vi "X DIM conditions.Facade.vi"(0 "Data In":T7, 2 "Display State In":T5, 3 "Container State":T6) -> (6 "Data Out":T7, 7 "Display State Out":T5, 8 "Action":T4)   [LabVIEW 2014, in "X DIM conditions.xctl"]
uses:
  X DIM conditions.xctl
  X DIM conditions.Data.ctl
  PTSequencer/PTSequencer.DIM service condition.ctl
  CSCore/CSSystem/CoreDefs/CoreDefs.rawDataType.ctl
  <vilib>/_xctls/Container State.ctl
  X DIM conditions.State.ctl
  <vilib>/_xctls/Action.ctl
  CSCore/CSSystem/CoreLib/CoreLib.string 2 byte array.vi
  CSCore/CSSystem/CoreLib/CoreLib.int 2 byte array.vi
  CSCore/CSSystem/CoreLib/CoreLib.int array 2 byte array.vi
  CSCore/CSSystem/CoreLib/CoreLib.short 2 byte array.vi
  CSCore/CSSystem/CoreLib/CoreLib.short array 2 byte array.vi
  CSCore/CSSystem/CoreLib/CoreLib.double 2 byte array.vi
  CSCore/CSSystem/CoreLib/CoreLib.double array 2 byte array.vi
  CSCore/CSSystem/CoreLib/CoreLib.float 2 byte array.vi
  CSCore/CSSystem/CoreLib/CoreLib.float array 2 byte array.vi
  <vilib>/_xctls/XControlSupport.lvlib
  CSCore/CSSystem/CoreLib/CoreLib.lvlib
  _common/PTUtils/PTUtils.lvlib
  CSlibraries/UtilityLib/UtilityLib.lvlib
  PTSequencer/PTSequencer.lvlib
panel:
  in  "element":T1
  in  "Scrollbar":i32(c297)
  in  "Control":T3
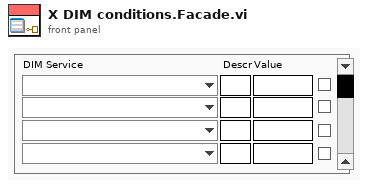
[diagram p1: front panel]
types:
  T1 = typedef "PTSequencer.lvlib/PTSequencer.DIM service condition.ctl" = cluster{"DIM service":string, "descr":string, "nomValue":T2, "actValue":T2, "matched":bool, "DIM Status":cluster{"no link":bool, "quality":i32, "Time Stamp":timestamp}}
  T2 = typedef "CoreDefs.rawDataType.ctl" = i8[]
  T3 = cluster{"Name 1":u16, "Descr 1":string, "Value 1":string, "Used 1":bool, "Name 2":u16, "Descr 2":string, "Value 2":string, "Used 2":bool, "Name 3":u16, "Descr 3":string, "Value 3":string, "Used 3":bool, "Name 4":u16, "Descr 4":string, "Value 4":string, "Used 4":bool}
  T4 = typedef "XControlSupport.lvlib/Action.ctl" = cluster{"Data Changed?":bool, "State Changed?":bool, "Action Name":string}
  T5 = typedef "X DIM conditions.xctl/X DIM conditions.State.ctl" = cluster{"index":i32}
  T6 = typedef "XControlSupport.lvlib/Container State.ctl" = cluster{"Indicator?":bool, "Run Mode?":bool, " Refnum":refnum<vi>}
  T7 = typedef "X DIM conditions.xctl/X DIM conditions.Data.ctl" = cluster{"DIM Services":string[], "data decsriptors":string[], "stop conditions":T1[]}
  T8 = enum8{"Enabled", "Disabled", "Disabled and Grayed Out"}
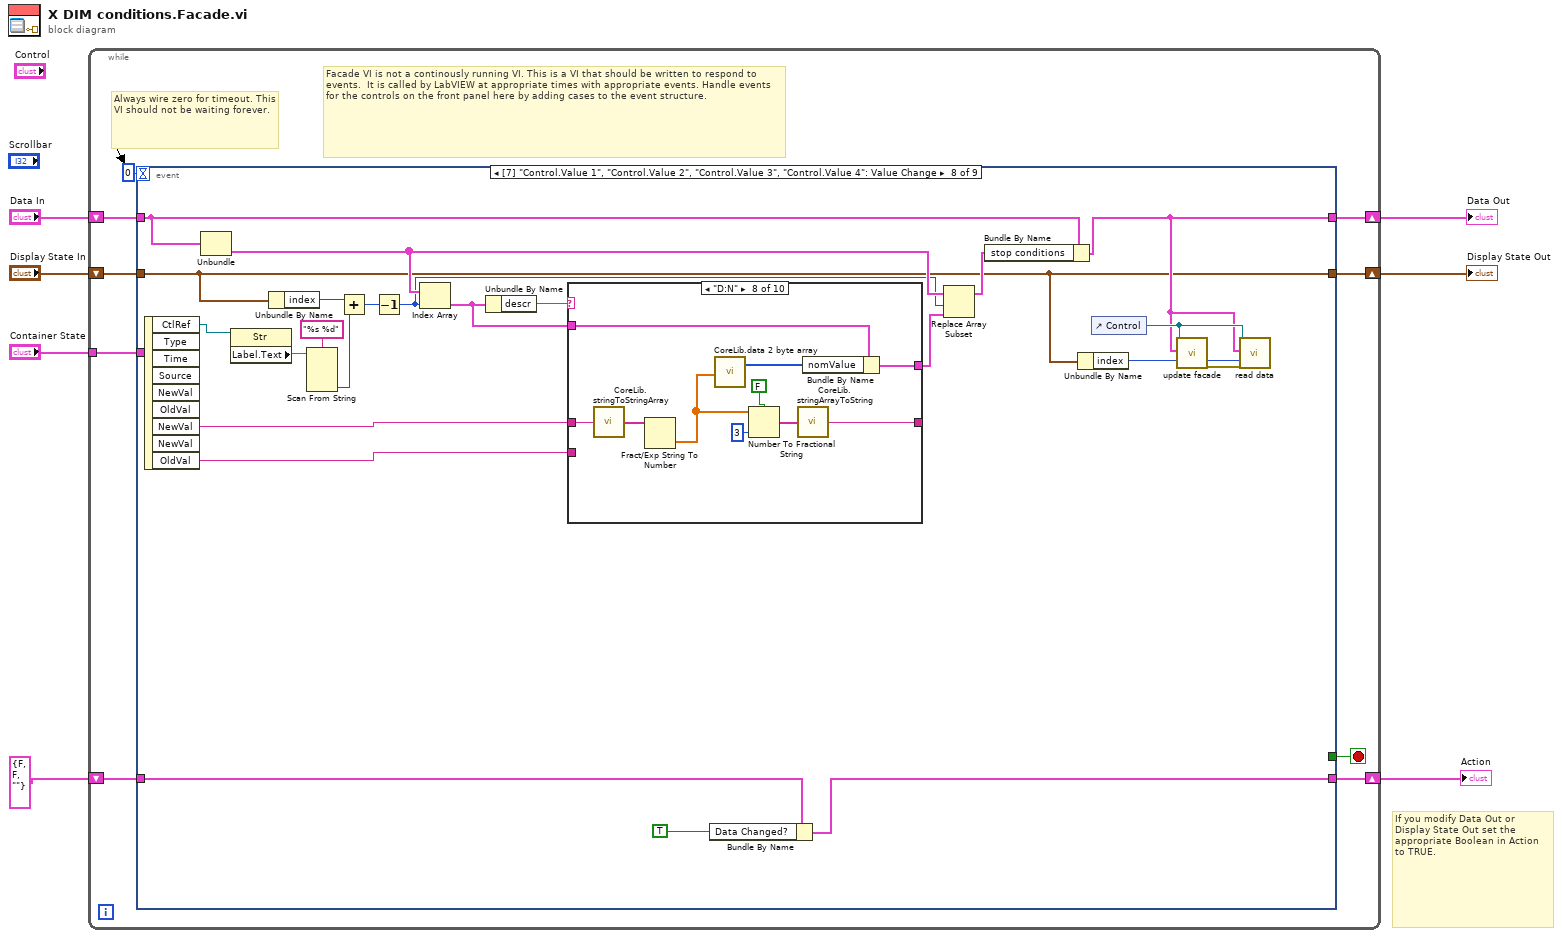
[diagram p0: block diagram]
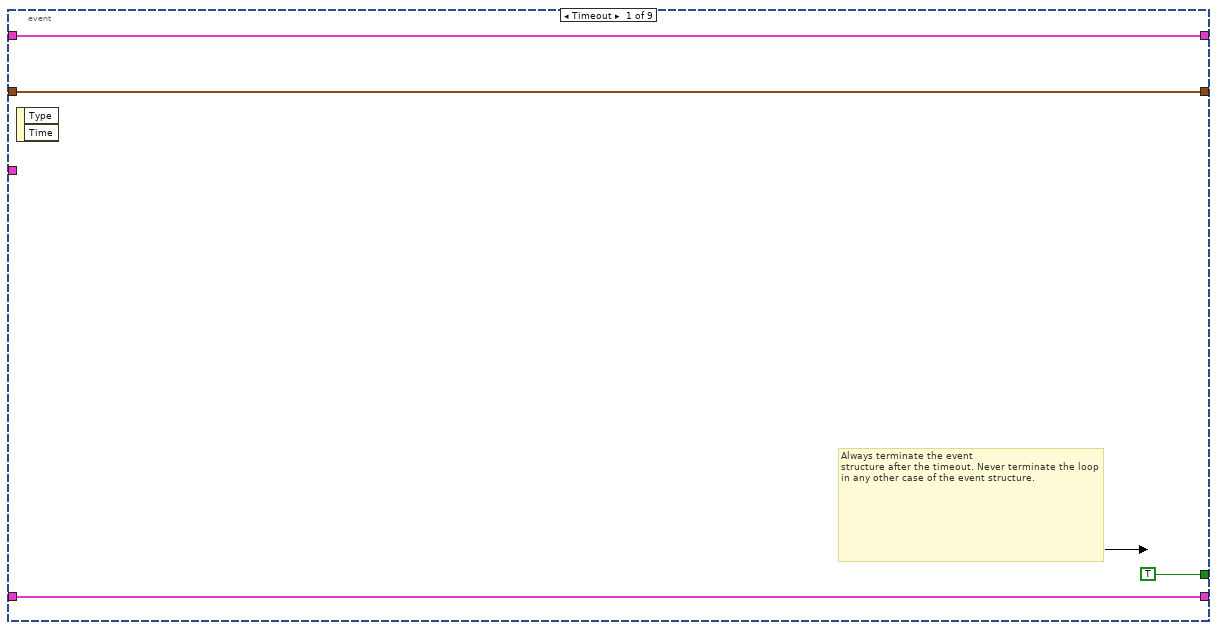
[diagram p2: hidden frame]
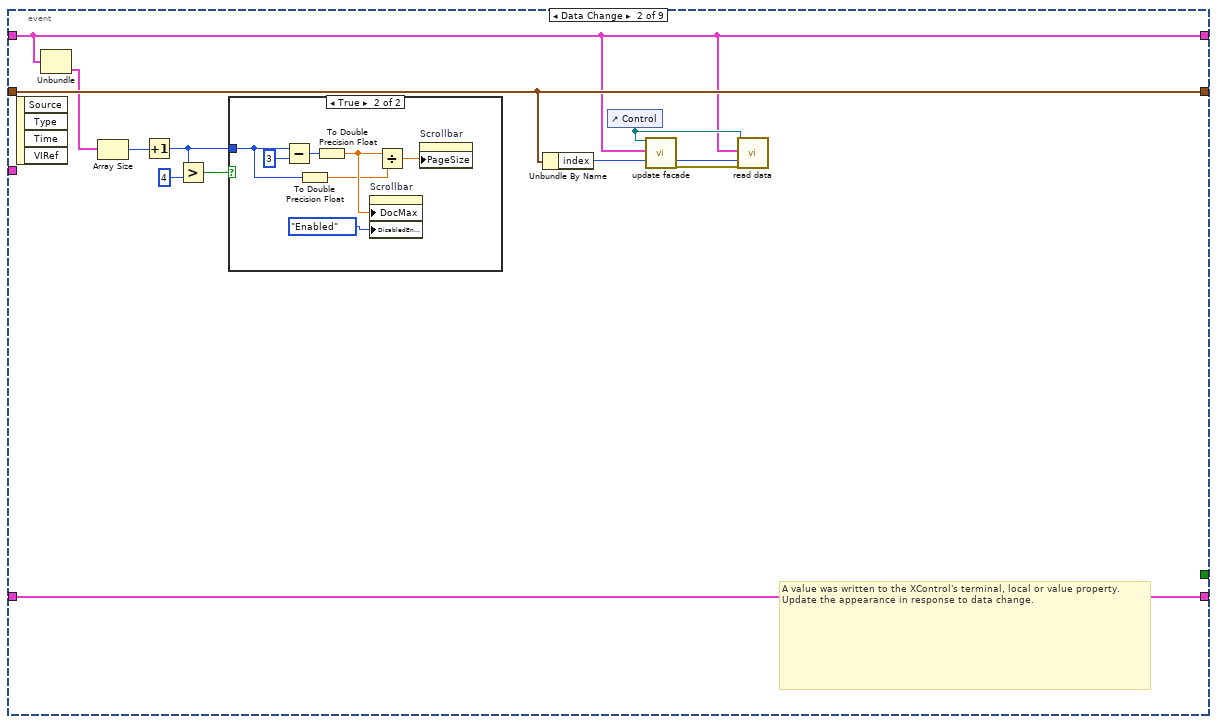
[diagram p3: hidden frame]
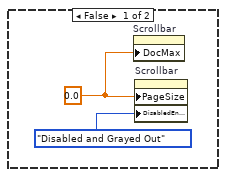
[diagram p4: hidden frame]
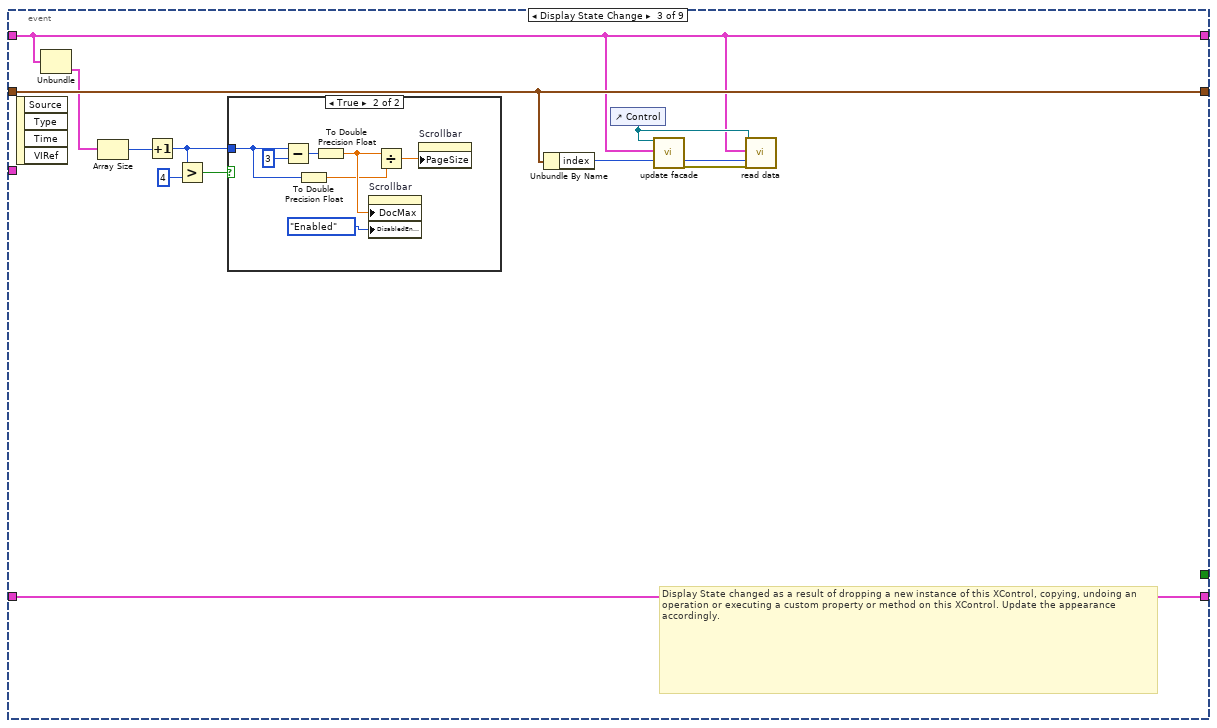
[diagram p5: hidden frame]
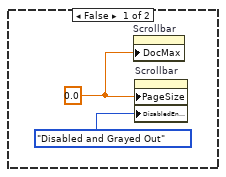
[diagram p6: hidden frame]
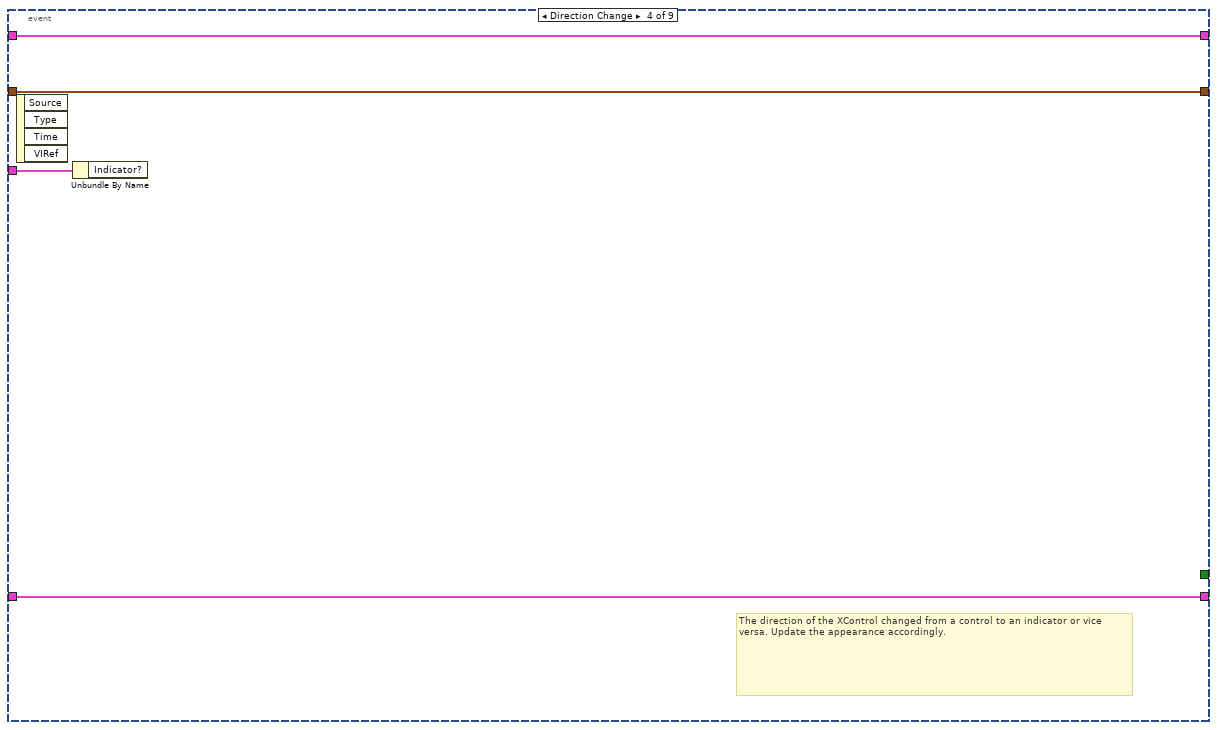
[diagram p7: hidden frame]
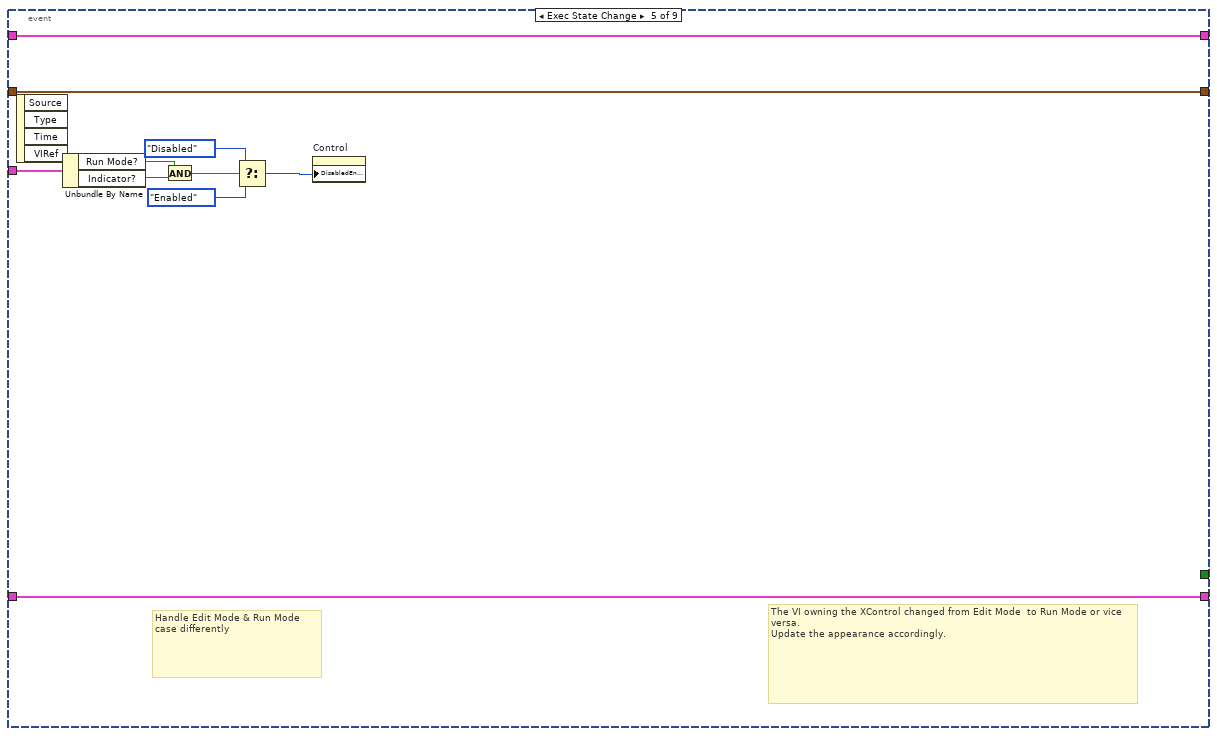
[diagram p8: hidden frame]
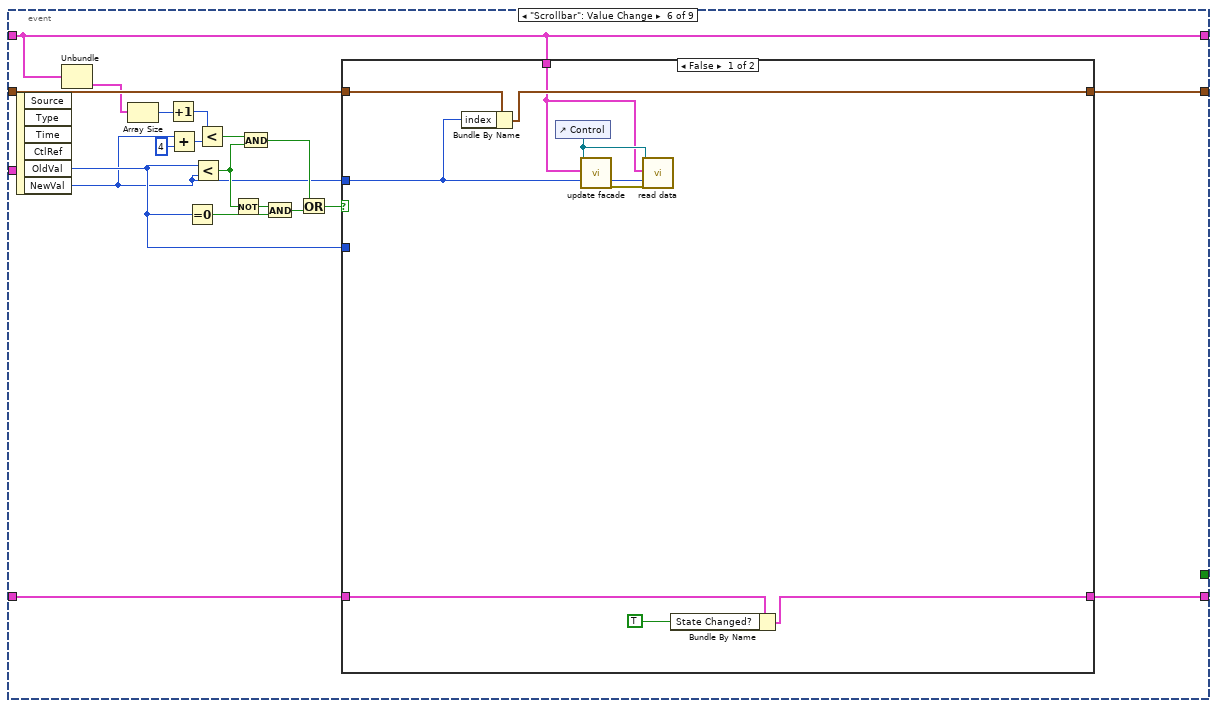
[diagram p9: hidden frame]
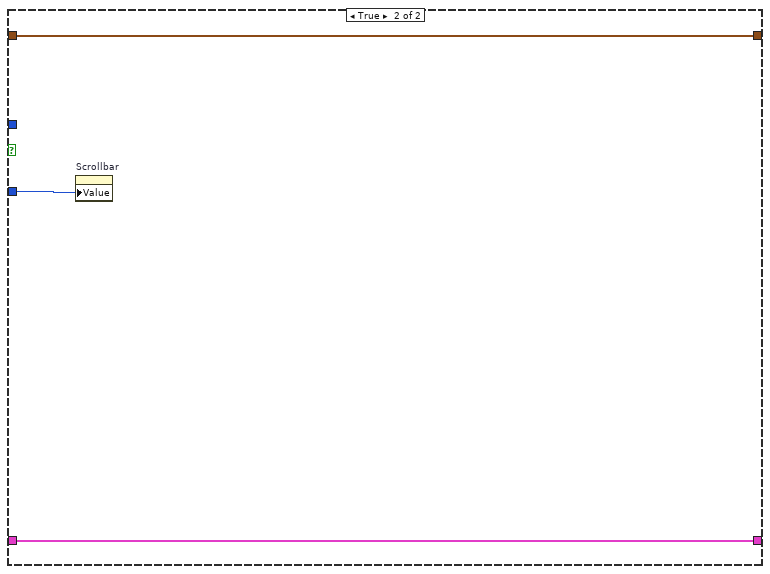
[diagram p10: hidden frame]
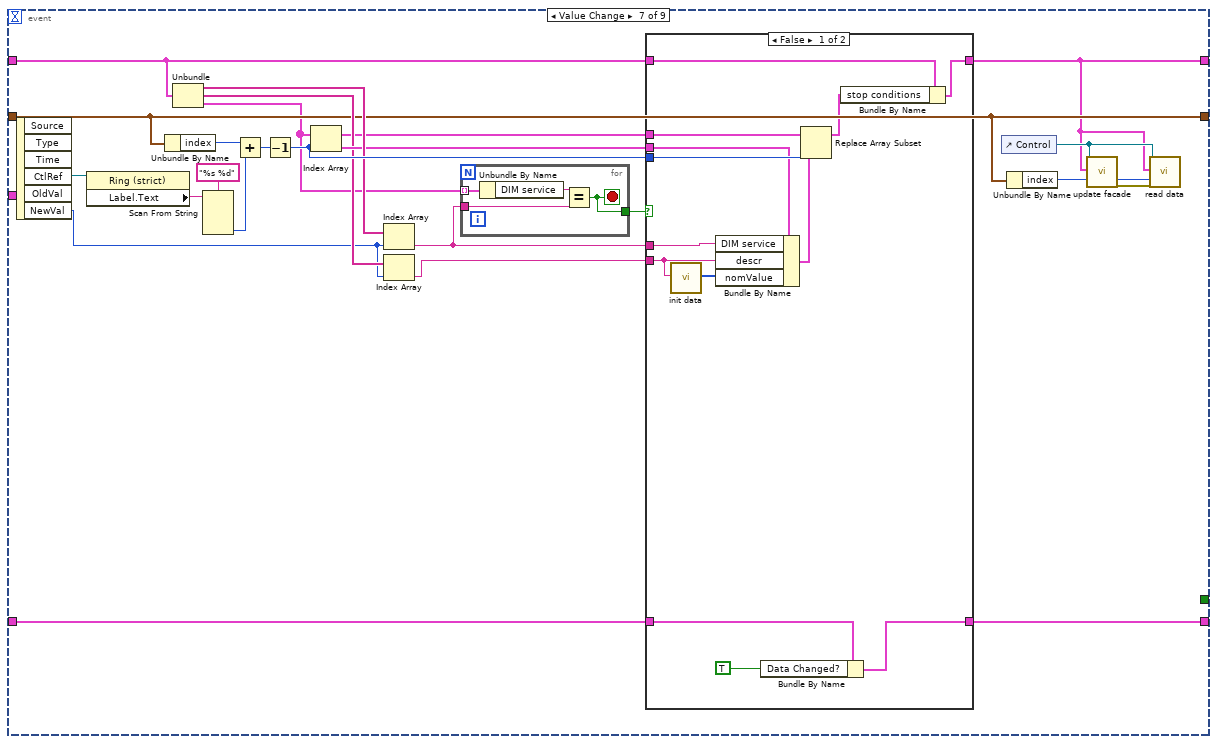
[diagram p11: hidden frame]
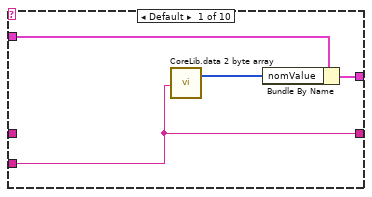
[diagram p13: hidden frame]
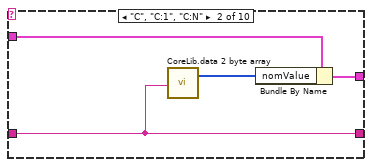
[diagram p14: hidden frame]
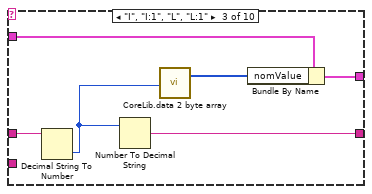
[diagram p15: hidden frame]
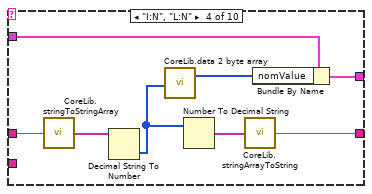
[diagram p16: hidden frame]
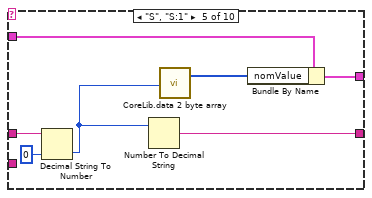
[diagram p17: hidden frame]
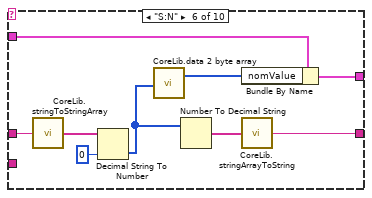
[diagram p18: hidden frame]
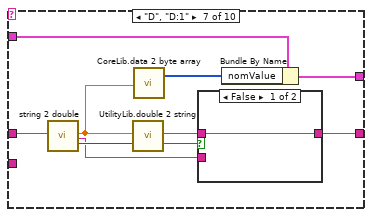
[diagram p19: hidden frame]
diagram:
  # "If you modify Data Out or\nDisplay State Out set the\nappropriate Boolean in Action\nto TRUE."
  n1 = while {
    shift-right: [w15] -> w4
    shift-left: "Display State In" -> [w16]
    tunnel: "Container State" -> [w12]
    shift-right: [w10] -> w7
    shift-left: "Data In" -> [w11]
    shift-right: [w8] -> w2
    shift-left: T4 {"Data Changed?"=FALSE, "State Changed?"=FALSE, "Action Name"=""} ("Action") -> [w9]
    stop <- w14 stop-if-true
    # "Facade VI is not a continously running VI. This is a VI that should be written to respond to events.  It is called by LabVIEW at appropriate times with appropriate events. Handle events for the controls on the front panel here by adding cases to the event structure."
    # "Always wire zero for timeout. This\nVI should not be waiting forever."
    n2 = event shown="[7] \"Control.Value 1\", \"Control.Value 2\", \"Control.Value 3\", \"Control.Value 4\": Value Change" {
      selector: _ -> [_ _ _ _ _ _ _ _ _]
      dyn-events: _ -> [_ _ _ _ _ _ _ _ _]
      timeout: 0 -> [_ _ _ _ _ _ _ _ _]
      tunnel: w16 -> [w18 w28 w48 w63 w73 w85 w113 w153 w259]
      tunnel: [w18 w28 w48 w63 w73 w83 w113 w153 w258] -> w15
      tunnel: [TRUE _ _ _ _ _ _ _ _] -> w14
      tunnel: w12 -> [_ _ _ w64 w74 _ _ _ _]
      tunnel: w11 -> [w17 w24 w45 w62 w72 w80 w121 w164 w269]
      tunnel: [w17 w24 w45 w62 w72 w80 w109 w154 w265] -> w10
      tunnel: [w19 w31 w51 w61 w71 w81 w114 w150 w256] -> w8
      tunnel: w9 -> [w19 w31 w51 w61 w71 w82 w115 w151 w257]
      event Timeout {
        # "Always terminate the event\nstructure after the timeout. Never terminate the loop in any other case of the event structure."
        n3 = event-data() -> ()  [unwired: 1 in, 2 out]
      }
      event Data Change {
        # "A value was written to the XControl's terminal, local or value property.\nUpdate the appearance in response to data change."
        n4 = event-data() -> ()  [unwired: 1 in, 4 out]
        n5 = Unbundle(w24) -> ("stop conditions"=w27:T1[])  [unwired: 2 out]
        n6 = Array Size(array=w27) -> (size(s)=w22:i32)
        n7 = Increment(x=w22) -> (x+1=w21:i32)
        n8 = Greater?(x=w21, y=4) -> (0:w29:bool)
        n9 = case shown="True" w29 {
          tunnel: w21 -> [_ w36]
          frame False {
            w32 = 0.0
            n10 = property on="Scrollbar" class="Scroll (strict)"("DocMax"=w32) -> ()  [unwired: 2 in, 2 out]
            n11 = property on="Scrollbar" class="Scroll (strict)"("PageSize"=w32, "DisabledEnum"=T8."Disabled and Grayed Out" ("Disabled")) -> ()  [unwired: 2 in, 2 out]
          }
          frame True {
            n12 = Subtract(x=w36, y=3) -> (x-y=w38:i32)
            n13 = To Double Precision Float(number=w36) -> (double precision float=w35:dbl)
            n14 = To Double Precision Float(number=w38) -> (double precision float=w37:dbl)
            n15 = property on="Scrollbar" class="Scroll (strict)"("DocMax"=w37, "DisabledEnum"=T8."Enabled" ("Disabled")) -> ()  [unwired: 2 in, 2 out]
            n16 = Divide(x=w37, y=w35) -> (x/y=w39:dbl)
            n17 = property on="Scrollbar" class="Scroll (strict)"("PageSize"=w39) -> ()  [unwired: 2 in, 2 out]
          }
        }
        n18 = Unbundle By Name(w28) -> ("index"=w23:i32)
        n19 = control-ref of="Control"() -> (w26:refnum<vi>)
        n20 = call "update facade.vi"("control ref"=w26, "Data In"=w24, "index"=w23) -> ("error out"=w25:errorcluster)  [unwired: 16 in]
        n21 = call "read data.vi"("Control ref"=w26, "Data In"=w24, "index"=w23, "error in (no error)"=w25) -> ()  [unwired: 16 in]
      }
      event Display State Change {
        # "Display State changed as a result of dropping a new instance of this XControl, copying, undoing an operation or executing a custom property or method on this XControl. Update the appearance accordingly."
        n22 = event-data() -> ()  [unwired: 1 in, 4 out]
        n23 = Unbundle(w45) -> ("stop conditions"=w47:T1[])  [unwired: 2 out]
        n24 = Array Size(array=w47) -> (size(s)=w42:i32)
        n25 = Increment(x=w42) -> (x+1=w41:i32)
        n26 = Greater?(x=w41, y=4) -> (0:w49:bool)
        n27 = case shown="True" w49 {
          tunnel: w41 -> [_ w56]
          frame False {
            w52 = 0.0
            n28 = property on="Scrollbar" class="Scroll (strict)"("DocMax"=w52) -> ()  [unwired: 2 in, 2 out]
            n29 = property on="Scrollbar" class="Scroll (strict)"("PageSize"=w52, "DisabledEnum"=T8."Disabled and Grayed Out" ("Disabled")) -> ()  [unwired: 2 in, 2 out]
          }
          frame True {
            n30 = Subtract(x=w56, y=3) -> (x-y=w58:i32)
            n31 = To Double Precision Float(number=w56) -> (double precision float=w55:dbl)
            n32 = To Double Precision Float(number=w58) -> (double precision float=w57:dbl)
            n33 = property on="Scrollbar" class="Scroll (strict)"("DocMax"=w57, "DisabledEnum"=T8."Enabled" ("Disabled")) -> ()  [unwired: 2 in, 2 out]
            n34 = Divide(x=w57, y=w55) -> (x/y=w59:dbl)
            n35 = property on="Scrollbar" class="Scroll (strict)"("PageSize"=w59) -> ()  [unwired: 2 in, 2 out]
          }
        }
        n36 = Unbundle By Name(w48) -> ("index"=w44:i32)
        n37 = control-ref of="Control"() -> (w46:refnum<vi>)
        n38 = call "update facade.vi"("control ref"=w46, "Data In"=w45, "index"=w44) -> ("error out"=w43:errorcluster)  [unwired: 16 in]
        n39 = call "read data.vi"("Control ref"=w46, "Data In"=w45, "index"=w44, "error in (no error)"=w43) -> ()  [unwired: 16 in]
      }
      event Direction Change {
        # "The direction of the XControl changed from a control to an indicator or vice versa. Update the appearance accordingly."
        n40 = event-data() -> ()  [unwired: 1 in, 4 out]
        n41 = Unbundle By Name(w64) -> ()  [unwired: 1 out]
      }
      event Exec State Change {
        # "The VI owning the XControl changed from Edit Mode  to Run Mode or vice versa.\nUpdate the appearance accordingly."
        # "Handle Edit Mode & Run Mode\ncase differently"
        n42 = event-data() -> ()  [unwired: 1 in, 4 out]
        n43 = Unbundle By Name(w74) -> ("Run Mode?"=w66:bool, "Indicator?"=w67:bool)
        n44 = And(x=w66, y=w67) -> (x .and. y?=w65:bool)
        n45 = Select(t=T8."Disabled" ("Disabled"), s=w65, f=T8."Enabled" ("Disabled")) -> (s? t:f=w68:T8)
        n46 = property on="Control" class="Clust (strict)"("DisabledEnum"=w68) -> ()  [unwired: 2 in, 2 out]
      }
      event "Scrollbar": Value Change {
        n47 = event-data() -> ("OldVal"=w84:i32, "NewVal"=w75:i32)  [unwired: 1 in, 4 out]
        n48 = Unbundle(w80) -> ("stop conditions"=w79:T1[])  [unwired: 2 out]
        n49 = Array Size(array=w79) -> (size(s)=w78:i32)
        n50 = Increment(x=w78) -> (x+1=w77:i32)
        n51 = Add(x=w75, y=4) -> (x+y=w92:i32)
        n52 = Equal To 0?(x=w84) -> (x = 0?=w88:bool)
        n53 = Less?(x=w84, y=w75) -> (x < y?=w89:bool)
        n54 = Less?(x=w77, y=w92) -> (x < y?=w91:bool)
        n55 = Not(x=w89) -> (.not. x?=w90:bool)
        n56 = And(x=w91, y=w89) -> (x .and. y?=w86:bool)
        n57 = And(x=w90, y=w88) -> (x .and. y?=w87:bool)
        n58 = Or(x=w86, y=w87) -> (x .or. y?=w76:bool)
        n59 = case shown="False" w76 {
          tunnel: w82 -> [w101 w105]
          tunnel: [w100 w105] -> w81
          tunnel: [w98 w104] -> w83
          tunnel: w85 -> [w99 w104]
          tunnel: w84 -> [_ w103]
          tunnel: w75 -> [w97 _]
          tunnel: w80 -> [w94 _]
          frame False {
            n60 = Bundle By Name(cluster=w99, "index"=w97) -> (w98:T5)
            n61 = control-ref of="Control"() -> (w95:refnum<vi>)
            n62 = call "update facade.vi"("control ref"=w95, "Data In"=w94, "index"=w97) -> ("error out"=w96:errorcluster)  [unwired: 16 in]
            n63 = call "read data.vi"("Control ref"=w95, "Data In"=w94, "index"=w97, "error in (no error)"=w96) -> ()  [unwired: 16 in]
            n64 = Bundle By Name(cluster=w101, "State Changed?"=TRUE) -> (w100:T4)
          }
          frame True {
            n65 = property on="Scrollbar" class="Scroll (strict)"("Value"=w103) -> ()  [unwired: 2 in, 2 out]
          }
        }
      }
      event "Control.Name 1", "Control.Name 2", "Control.Name 3", "Control.Name 4": Value Change {
        n66 = event-data() -> ("CtlRef"=w123:refnum<vi>, "NewVal"=w117:u16)  [unwired: 1 in, 4 out]
        n67 = property class="Ring (strict)"(reference=w123) -> ("Label.Text"=w128:string)  [unwired: 1 in, 2 out]
        n68 = Unbundle By Name(w113) -> ("index"=w126:i32)
        n69 = Unbundle(w121) -> ("DIM Services"=w120:string[], "data decsriptors"=w118:string[], "stop conditions"=w108:T1[])
        n70 = Scan From String(format string="%s %d", input string=w128) -> (output 2=w124:i32)  [unwired: 5 in, 3 out]
        n71 = Add(x=w126, y=w124) -> (x+y=w125:i32)
        n72 = Decrement(x=w125) -> (x-1=w122:i32)
        n73 = Index Array(array=w108, index=w122) -> (element=w119:T1)
        n74 = Index Array(array=w120, index=w117) -> (element=w107:string)
        n75 = Index Array(array=w118, index=w117) -> (element=w116:string)
        n76 = for {
          tunnel: w108 -> [w147] mode=indexing
          tunnel: w107 -> [w145]
          tunnel: [w144] -> w106
          stop <- w144 stop-if-true
          n77 = Unbundle By Name(w147) -> ("DIM service"=w146:string)
          n78 = Equal?(x=w146, y=w145) -> (x = y?=w144:bool)
        }
        n79 = case shown="False" w106 {
          tunnel: w122 -> [w141 _]
          tunnel: w121 -> [w140 w143]
          tunnel: w119 -> [w139 _]
          tunnel: w116 -> [w129 _]
          tunnel: w115 -> [w135 w142]
          tunnel: [w134 w142] -> w114
          tunnel: [w133 w143] -> w109
          tunnel: w108 -> [w132 _]
          tunnel: w107 -> [w131 _]
          frame False {
            n80 = call "init data.vi"("descr"=w129) -> ("nomValue"=w130:T2)  [unwired: 18 in]
            n81 = Bundle By Name(cluster=w139, "DIM service"=w131, "descr"=w129, "nomValue"=w130) -> (w138:T1)
            n82 = Bundle By Name(cluster=w135, "Data Changed?"=TRUE) -> (w134:T4)
            n83 = Replace Array Subset(array=w132, new element=w138, index=w141) -> (w137:T1[])
            n84 = Bundle By Name(cluster=w140, "stop conditions"=w137) -> (w133:T7)
          }
          frame True {
          }
        }
        n85 = control-ref of="Control"() -> (w112:refnum<vi>)
        n86 = Unbundle By Name(w113) -> ("index"=w111:i32)
        n87 = call "update facade.vi"("control ref"=w112, "Data In"=w109, "index"=w111) -> ("error out"=w110:errorcluster)  [unwired: 16 in]
        n88 = call "read data.vi"("Control ref"=w112, "Data In"=w109, "index"=w111, "error in (no error)"=w110) -> ()  [unwired: 16 in]
      }
      event "Control.Value 1", "Control.Value 2", "Control.Value 3", "Control.Value 4": Value Change {
        n89 = event-data() -> ("CtlRef"=w166:refnum<vi>, "NewVal"=w157:string, "OldVal"=w163:string)  [unwired: 1 in, 6 out]
        n90 = Unbundle(w164) -> ("stop conditions"=w162:T1[])  [unwired: 2 out]
        n91 = property class="Str"(reference=w166) -> ("Label.Text"=w170:string)  [unwired: 1 in, 2 out]
        n92 = Unbundle By Name(w153) -> ("index"=w168:i32)
        n93 = Scan From String(format string="%s %d", input string=w170) -> (output 2=w148:i32)  [unwired: 5 in, 3 out]
        n94 = Add(x=w168, y=w148) -> (x+y=w167:i32)
        n95 = Decrement(x=w167) -> (x-1=w161:i32)
        n96 = Index Array(array=w162, index=w161) -> (element=w160:T1)
        n97 = Unbundle By Name(w160) -> ("descr"=w165:string)
        n98 = case shown="\"D:N\"" w165 {
          tunnel: w163 -> [w171 _ _ _ _ _ _ _ _ _]
          tunnel: w160 -> [w174 w178 w181 w189 w197 w205 w216 w227 w240 w252]
          tunnel: [w173 w177 w182 w188 w196 w204 w215 w226 w239 w251] -> w159
          tunnel: w157 -> [_ w175 w184 w192 w198 w206 w218 w229 w241 w253]
          tunnel: [w171 w175 w179 w185 w193 w201 w209 w222 w236 w247] -> _
          frame Default {
            n99 = call-poly "CoreLib.data 2 byte array.vi"("string"=w171) -> ("byteArray out"=w172:T2)  [unwired: 18 in]
            n100 = Bundle By Name(cluster=w174, "nomValue"=w172) -> (w173:T1)
          }
          frame "C", "C:1", "C:N" {
            n101 = call-poly "CoreLib.data 2 byte array.vi"("string"=w175) -> ("byteArray out"=w176:T2)  [unwired: 18 in]
            n102 = Bundle By Name(cluster=w178, "nomValue"=w176) -> (w177:T1)
          }
          frame "I", "I:1", "L", "L:1" {
            n103 = Decimal String To Number(string=w184) -> (number=w180:i32)  [unwired: 2 in, 1 out]
            n104 = Number To Decimal String(number=w180) -> (decimal integer string=w179:string)  [unwired: 1 in]
            n105 = call-poly "CoreLib.data 2 byte array.vi"("i32"=w180) -> ("byteArray out"=w183:T2)  [unwired: 18 in]
            n106 = Bundle By Name(cluster=w181, "nomValue"=w183) -> (w182:T1)
          }
          frame "I:N", "L:N" {
            n107 = call "CoreLib.stringToStringArray.vi"("String"=w192) -> ("Array"=w191:string[])
            n108 = Decimal String To Number(string=w191) -> (number=w187:i32[])  [unwired: 2 in, 1 out]
            n109 = call-poly "CoreLib.data 2 byte array.vi"("[i32]"=w187) -> ("byteArray out"=w190:T2)  [unwired: 18 in]
            n110 = Number To Decimal String(number=w187) -> (decimal integer string=w186:string[])  [unwired: 1 in]
            n111 = call "CoreLib.stringArrayToString.vi"("Array"=w186) -> ("String"=w185:string)
            n112 = Bundle By Name(cluster=w189, "nomValue"=w190) -> (w188:T1)
          }
          frame "S", "S:1" {
            n113 = Decimal String To Number(string=w198, default (0L)=i16 0 ("default (0 I32)")) -> (number=w194:i16)  [unwired: 1 in, 1 out]
            n114 = Number To Decimal String(number=w194) -> (decimal integer string=w193:string)  [unwired: 1 in]
            n115 = call-poly "CoreLib.data 2 byte array.vi"("i16"=w194) -> ("byteArray out"=w199:T2)  [unwired: 18 in]
            n116 = Bundle By Name(cluster=w197, "nomValue"=w199) -> (w196:T1)
          }
          frame "S:N" {
            n117 = call "CoreLib.stringToStringArray.vi"("String"=w206) -> ("Array"=w208:string[])
            n118 = Decimal String To Number(string=w208, default (0L)=i16 0 ("default (0 I32)")) -> (number=w200:i16[])  [unwired: 1 in, 1 out]
            n119 = call-poly "CoreLib.data 2 byte array.vi"("[i16]"=w200) -> ("byteArray out"=w207:T2)  [unwired: 18 in]
            n120 = Number To Decimal String(number=w200) -> (decimal integer string=w202:string[])  [unwired: 1 in]
            n121 = Bundle By Name(cluster=w205, "nomValue"=w207) -> (w204:T1)
            n122 = call "CoreLib.stringArrayToString.vi"("Array"=w202) -> ("String"=w201:string)
          }
          frame "D", "D:1" {
            n123 = call "string 2 double.vi"("string"=w218) -> ("number"=w213:dbl, "scanned string"=w210:string, "length"=w214:u8)  [unwired: 15 in, 1 out]
            n124 = call "UtilityLib.double 2 string.vi"("Numeric"=w213, "length"=w214) -> ("String"=w211:string, "loss free"=w212:bool)  [unwired: 16 in]
            n125 = call-poly "CoreLib.data 2 byte array.vi"("f64"=w213) -> ("byteArray out"=w217:T2)  [unwired: 18 in]
            n126 = case shown="False" w212 {
              tunnel: w211 -> [w219 _]
              tunnel: w210 -> [_ w220]
              tunnel: [w219 w220] -> w209
              frame False {
              }
              frame True {
              }
            }
            n127 = Bundle By Name(cluster=w216, "nomValue"=w217) -> (w215:T1)
          }
          frame "D:N" {
            n128 = call "CoreLib.stringToStringArray.vi"("String"=w229) -> ("Array"=w228:string[])
            n129 = Fract/Exp String To Number(string=w228) -> (number=w223:dbl[])  [unwired: 3 in, 1 out]
            n130 = call-poly "CoreLib.data 2 byte array.vi"("[d64]"=w223) -> ("byteArray out"=w230:T2)  [unwired: 18 in]
            n131 = Number To Fractional String(use system decimal point (T)=FALSE, number=w223, precision (6)=i16 3) -> (F-format string=w224:string[])  [unwired: 1 in]
            n132 = call "CoreLib.stringArrayToString.vi"("Array"=w224) -> ("String"=w222:string)
            n133 = Bundle By Name(cluster=w227, "nomValue"=w230) -> (w226:T1)
          }
          frame "F", "F:1" {
            n134 = call "string 2 double.vi"("string"=w241) -> ("number"=w233:dbl, "scanned string"=w235:string, "length"=w234:u8)  [unwired: 15 in, 1 out]
            n135 = To Single Precision Float(number=w233) -> (single precision float=w232:sgl)
            n136 = To Double Precision Float(number=w232) -> (double precision float=w231:dbl)
            n137 = call "UtilityLib.double 2 string.vi"("Numeric"=w231, "length"=w234) -> ("String"=w237:string, "loss free"=w238:bool)  [unwired: 16 in]
            n138 = call-poly "CoreLib.data 2 byte array.vi"("f32"=w232) -> ("byteArray out"=w242:T2)  [unwired: 18 in]
            n139 = case shown="False" w238 {
              tunnel: w237 -> [w243 _]
              tunnel: w235 -> [_ w244]
              tunnel: [w243 w244] -> w236
              frame False {
              }
              frame True {
              }
            }
            n140 = Bundle By Name(cluster=w240, "nomValue"=w242) -> (w239:T1)
          }
          frame "F:N" {
            n141 = call "CoreLib.stringToStringArray.vi"("String"=w253) -> ("Array"=w254:string[])
            n142 = Fract/Exp String To Number(string=w254) -> (number=w246:dbl[])  [unwired: 3 in, 1 out]
            n143 = To Single Precision Float(number=w246) -> (single precision float=w250:sgl[])
            n144 = Number To Fractional String(use system decimal point (T)=FALSE, number=w246, precision (6)=i16 3) -> (F-format string=w248:string[])  [unwired: 1 in]
            n145 = call-poly "CoreLib.data 2 byte array.vi"("[f32]"=w250) -> ("byteArray out"=w255:T2)  [unwired: 18 in]
            n146 = call "CoreLib.stringArrayToString.vi"("Array"=w248) -> ("String"=w247:string)
            n147 = Bundle By Name(cluster=w252, "nomValue"=w255) -> (w251:T1)
          }
        }
        n148 = Bundle By Name(cluster=w151, "Data Changed?"=TRUE) -> (w150:T4)
        n149 = Replace Array Subset(array=w162, new element=w159, index=w161) -> (w158:T1[])
        n150 = Bundle By Name(cluster=w164, "stop conditions"=w158) -> (w154:T7)
        n151 = Unbundle By Name(w153) -> ("index"=w152:i32)
        n152 = control-ref of="Control"() -> (w156:refnum<vi>)
        n153 = call "update facade.vi"("control ref"=w156, "Data In"=w154, "index"=w152) -> ("error out"=w155:errorcluster)  [unwired: 16 in]
        n154 = call "read data.vi"("Control ref"=w156, "Data In"=w154, "index"=w152, "error in (no error)"=w155) -> ()  [unwired: 16 in]
      }
      event "Control.Used 1", "Control.Used 2", "Control.Used 3", "Control.Used 4": Value Change {
        n155 = event-data() -> ("CtlRef"=w275:refnum<vi>, "NewVal"=w274:bool)  [unwired: 1 in, 1 out]
        n156 = property class="Bool (strict)"(reference=w275) -> ("Label.Text"=w280:string)  [unwired: 1 in, 2 out]
        n157 = Unbundle(w269) -> ("DIM Services"=w271:string[], "data decsriptors"=w270:string[], "stop conditions"=w273:T1[])
        n158 = Unbundle By Name(w259) -> ("index"=w278:i32)
        n159 = Scan From String(format string="%s %d", input string=w280) -> (output 2=w276:i32)  [unwired: 5 in, 3 out]
        n160 = Add(x=w278, y=w276) -> (x+y=w277:i32)
        n161 = Decrement(x=w277) -> (x-1=w272:i32)
        n162 = case shown="True" w274 {
          tunnel: w273 -> [w305 w326]
          tunnel: w272 -> [w304 _]
          tunnel: [w303 w328] -> w262
          tunnel: w271 -> [_ w325]
          tunnel: w270 -> [_ w323]
          tunnel: w259 -> [w299 w327]
          tunnel: [w298 w327] -> w258
          tunnel: w257 -> [w295 w319]
          tunnel: [w294 w318] -> w256
          frame False {
            n163 = Delete From Array(array=w305, index=w304) -> (array with subset deleted=w303:T1[])  [unwired: 1 in, 1 out]
            n164 = Unbundle By Name(w299) -> ("index"=w296:i32)
            n165 = Array Size(array=w303) -> (size(s)=w302:i32)
            n166 = Increment(x=w302) -> (x+1=w300:i32)
            n167 = Add(x=4, y=w296) -> (x+y=w301:i32)
            n168 = Decrement(x=w296) -> (x-1=w293:i32)
            n169 = Less?(x=w300, y=w301) -> (x < y?=w291:bool)
            n170 = Greater Or Equal To 0?(x=w293) -> (x >= 0?=w292:bool)
            n171 = And(x=w291, y=w292) -> (x .and. y?=w290:bool)
            n172 = case shown="True" w290 {
              tunnel: w299 -> [w309 w316]
              tunnel: [w309 w317] -> w298
              tunnel: w293 -> [_ w315]
              tunnel: w295 -> [w307 w314]
              tunnel: [w306 w313] -> w294
              frame False {
                n173 = Bundle By Name(cluster=w307, "Data Changed?"=TRUE) -> (w306:T4)
              }
              frame True {
                w312 = TRUE ("Data Changed?")
                n174 = property on="Scrollbar" class="Scroll (strict)"() -> ("Value"=w310:i32)  [unwired: 2 in, 2 out]
                n175 = Bundle By Name(cluster=w316, "index"=w315) -> (w317:T5)
                n176 = Bundle By Name(cluster=w314, "Data Changed?"=w312, "State Changed?"=w312) -> (w313:T4)
                n177 = Decrement(x=w310) -> (x-1=w311:i32)
                n178 = property on="Scrollbar" class="Scroll (strict)"("Value"=w311) -> ()  [unwired: 2 in, 2 out]
              }
            }
          }
          frame True {
            n179 = for {
              tunnel: w326 -> [w347] mode=indexing
              tunnel: [w346] -> w324 mode=indexing
              n180 = Unbundle By Name(w347) -> ("DIM service"=w346:string)
            }
            n181 = for {
              tunnel: w325 -> [w342] mode=indexing
              tunnel: w324 -> [w345]
              tunnel: w323 -> [w341] mode=indexing
              tunnel: [w343] -> w322
              tunnel: [w342] -> w321
              tunnel: [w341] -> w320
              stop <- w343 stop-if-true
              n182 = Search 1D Array(1D array=w345, element=w342) -> (index of element=w344:i32)  [unwired: 1 in]
              n183 = Less Than 0?(x=w344) -> (x < 0?=w343:bool)
            }
            n184 = case shown="True" w322 {
              tunnel: [w330 w338] -> w328
              tunnel: w326 -> [w330 w337]
              tunnel: w321 -> [_ w336]
              tunnel: w320 -> [_ w331]
              tunnel: w319 -> [w329 w334]
              tunnel: [w329 w333] -> w318
              frame False {
              }
              frame True {
                n185 = call "init data.vi"("descr"=w331) -> ("nomValue"=w332:T2)  [unwired: 18 in]
                n186 = Bundle By Name(cluster=w334, "Data Changed?"=TRUE) -> (w333:T4)
                n187 = Bundle By Name(cluster="element", "DIM service"=w336, "descr"=w331, "nomValue"=w332) -> (w339:T1)
                n188 = Build Array (concatenate)(w337, w339) -> (w338:T1[])
              }
            }
          }
        }
        n189 = Bundle By Name(cluster=w269, "stop conditions"=w262) -> (w265:T7)
        n190 = Array Size(array=w262) -> (size(s)=w261:i32)
        n191 = Increment(x=w261) -> (x+1=w260:i32)
        n192 = Greater?(x=w260, y=4) -> (0:w263:bool)
        n193 = case shown="True" w263 {
          tunnel: w260 -> [_ w283]
          frame False {
            w281 = 0.0
            n194 = property on="Scrollbar" class="Scroll (strict)"("DocMax"=w281) -> ()  [unwired: 2 in, 2 out]
            n195 = property on="Scrollbar" class="Scroll (strict)"("PageSize"=w281, "DisabledEnum"=T8."Disabled and Grayed Out" ("Disabled")) -> ()  [unwired: 2 in, 2 out]
          }
          frame True {
            n196 = Subtract(x=w283, y=3) -> (x-y=w288:i32)
            n197 = To Double Precision Float(number=w283) -> (double precision float=w286:dbl)
            n198 = To Double Precision Float(number=w288) -> (double precision float=w287:dbl)
            n199 = property on="Scrollbar" class="Scroll (strict)"("DocMax"=w287, "DisabledEnum"=T8."Enabled" ("Disabled")) -> ()  [unwired: 2 in, 2 out]
            n200 = Divide(x=w287, y=w286) -> (x/y=w289:dbl)
            n201 = property on="Scrollbar" class="Scroll (strict)"("PageSize"=w289) -> ()  [unwired: 2 in, 2 out]
          }
        }
        n202 = Unbundle By Name(w258) -> ("index"=w266:i32)
        n203 = control-ref of="Control"() -> (w268:refnum<vi>)
        n204 = call "update facade.vi"("control ref"=w268, "Data In"=w265, "index"=w266) -> ("error out"=w267:errorcluster)  [unwired: 16 in]
        n205 = call "read data.vi"("Control ref"=w268, "Data In"=w265, "index"=w266, "error in (no error)"=w267) -> ()  [unwired: 16 in]
      }
    }
  }
  "Display State Out" <- w4
  "Data Out" <- w7
  "Action" <- w2
